vi "鼠标获取曲线值 - 副本.vi"(9 "鼠标坐标":T1, 10 "图谱引用":refnum<vi>, 11 "字符引用":refnum<vi>) -> ()   [LabVIEW 2020]
uses:
  <vilib>/Utility/miscctls.llb/LVPoint32TypeDef.ctl
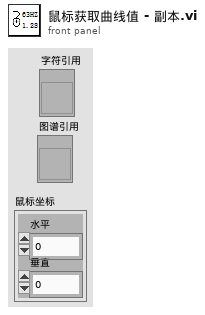
[diagram p1: front panel]
types:
  T1 = typedef "LVPoint32TypeDef.ctl" = cluster{"Horizontal":i32, "Vertical":i32}
  T2 = typedef "LVPointDoubleTypeDef.ctl" = cluster{"Cursor X":dbl, "Cursor Y":dbl}
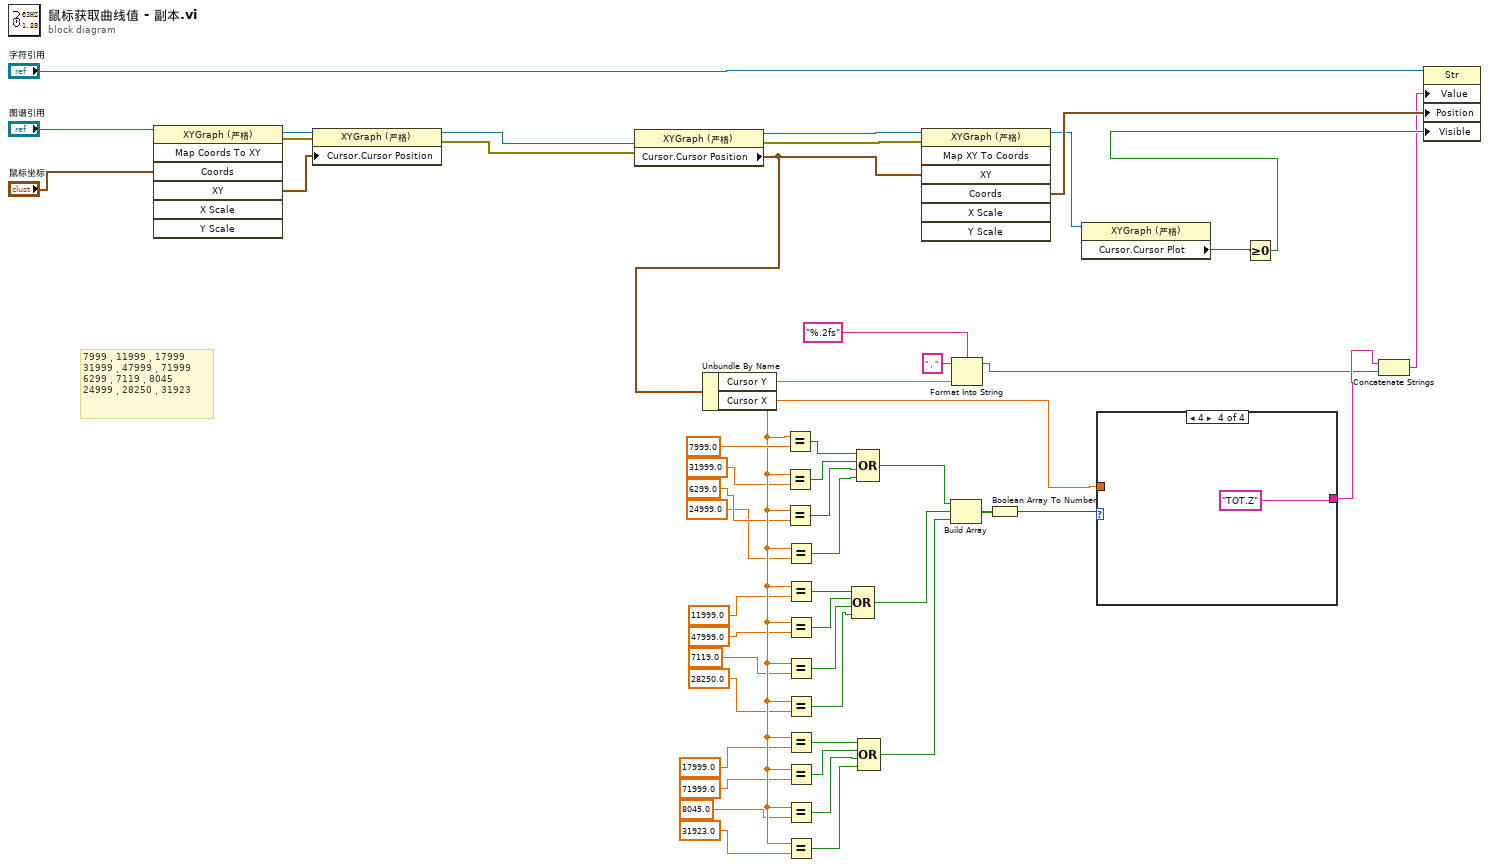
[diagram p0: block diagram]
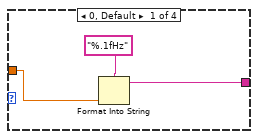
[diagram p2: hidden frame]
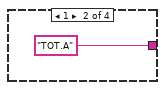
[diagram p3: hidden frame]
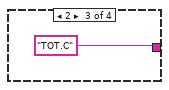
[diagram p4: hidden frame]
diagram:
  # "7999，11999，17999\n31999，47999，71999\n6299，7119，8045\n24999，28250，31923"
  n1 = invoke class="XYGraph (严格)" method="Map Coords To XY"(reference="图谱引用", "Coords"="鼠标坐标") -> (reference out=w49:refnum<vi>, error out=w48:errorcluster, "XY"=w47:cluster{"X":dbl, "Y":dbl})  [unwired: 5 in, 4 out]
  n2 = property class="XYGraph (严格)"(reference=w49, error in=w48, "Cursor.Cursor Position"=w47) -> (reference out=w41:refnum<vi>, error out=w43:errorcluster)
  n3 = property class="XYGraph (严格)"(reference=w41, error in=w43) -> (reference out=w45:refnum<vi>, error out=w44:errorcluster, "Cursor.Cursor Position"=w4:T2)
  n4 = Unbundle By Name(w4) -> ("Cursor Y"=w37:dbl, "Cursor X"=w20:dbl)
  n5 = Equal?(x=w20, y=7999.0) -> (x = y?=w35:bool)
  n6 = Equal?(x=w20, y=31999.0) -> (x = y?=w34:bool)
  n7 = Equal?(x=w20, y=6299.0) -> (x = y?=w33:bool)
  n8 = Equal?(x=w20, y=24999.0) -> (x = y?=w23:bool)
  n9 = Equal?(x=w20, y=11999.0) -> (x = y?=w32:bool)
  n10 = Equal?(x=w20, y=47999.0) -> (x = y?=w31:bool)
  n11 = Equal?(x=w20, y=7119.0) -> (x = y?=w22:bool)
  n12 = Equal?(x=w20, y=28250.0) -> (x = y?=w21:bool)
  n13 = Equal?(x=w20, y=17999.0) -> (x = y?=w30:bool)
  n14 = Equal?(x=w20, y=71999.0) -> (x = y?=w8:bool)
  n15 = Equal?(x=w20, y=8045.0) -> (x = y?=w7:bool)
  n16 = Equal?(x=w20, y=31923.0) -> (x = y?=w6:bool)
  n17 = Compound Arithmetic op=OR ("复合运算")(w32, w31, w22, w21) -> (w28:bool)
  n18 = Compound Arithmetic op=OR ("复合运算")(w35, w34, w33, w23) -> (w29:bool)
  n19 = Compound Arithmetic op=OR ("复合运算")(w30, w8, w7, w6) -> (w27:bool)
  n20 = invoke class="XYGraph (严格)" method="Map XY To Coords"(reference=w45, error in=w44, "XY"=w4) -> (reference out=w40:refnum<vi>, "Coords"=w46:T1)  [unwired: 4 in, 5 out]
  n21 = Build Array(w29, w28, w27) -> (w26:bool[])
  n22 = Format Into String(format string="%.2fs" ("格式字符串"), initial string="，" ("初始字符串"), w37) -> (resulting string=w2:string)  [unwired: 1 in, 1 out]
  n23 = Boolean Array To Number(Boolean array=w26) -> (number=w25:u32)
  n24 = property class="XYGraph (严格)"(reference=w40) -> ("Cursor.Cursor Plot"=w39:i32)  [unwired: 1 in, 2 out]
  n25 = case shown="4" w25 {
    tunnel: w20 -> [w54 _ _ _]
    tunnel: [w52 "TOT.A" ("格式字符串") "TOT.C" ("格式字符串") "TOT.Z" ("格式字符串")] -> w3
    frame 0, Default {
      n26 = Format Into String(format string="%.1fHz" ("格式字符串"), w54) -> (resulting string=w52:string)  [unwired: 2 in, 1 out]
    }
    frame 1 {
    }
    frame 2 {
    }
    frame 4 {
    }
  }
  n27 = Greater Or Equal To 0?(x=w39) -> (x >= 0?=w38:bool)
  n28 = Concatenate Strings(w3, w2) -> (w5:string)
  n29 = property class="Str"(reference="字符引用", "Value"=w5, "Position"=w46, "Visible"=w38) -> ()  [unwired: 1 in, 2 out]
